vi "Get Local Chassis Modules References.vi"(8 "error in":errorcluster, 11 "Local Chassis Reference In":T1 format="%.0x") -> (0 "error out":errorcluster, 1 "Modules Found":bool, 2 "Modules References":T1[](array[typedef]) format="%.0x", 3 "Local Chassis Reference Out":T1 format="%.0x")   [LabVIEW 2017, in "Scan Engine Custom Device.lvlib"]
uses:
  Scan Engine Custom Device.lvlib
  <vilib>/NI Veristand/Custom Device API/Custom Device Item Ref.ctl
  Globals/Scan Engine GUIDs.vi
  <vilib>/NI Veristand/Custom Device Tools/Custom Device Utility Library/NI VeriStand - Search for All Items by GUID.vi
  <vilib>/NI Veristand/Custom Device Tools/Custom Device Utility Library/Custom Device Utility Library.lvlib
  <vilib>/NI Veristand/Custom Device API/Custom Device API.lvlib
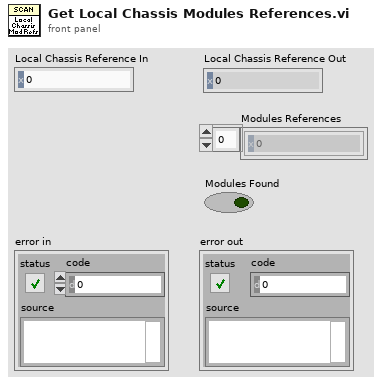
[diagram p1: front panel]
types:
  T1 = typedef "Custom Device API.lvlib/Custom Device Item Ref.ctl" = u64
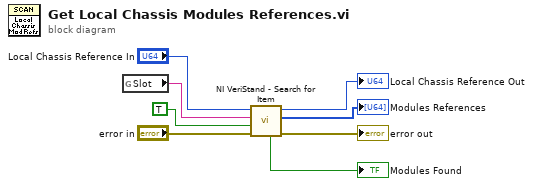
[diagram p0: block diagram]
diagram:
  n1 = global read "Scan Engine GUIDs.vi" "Slot"() -> (w8:string)
  n2 = call-poly <vilib>:"NI VeriStand - Search for Item.vi"("error in"="error in", "Find All? (T)"=TRUE, "Item GUID"=w8, "Section Ref in"="Local Chassis Reference In") -> ("error out"=→"error out":errorcluster, "Item Refs"=→"Modules References":T1[], "Section Ref out"=→"Local Chassis Reference Out":T1, "Found"=→"Modules Found":bool)  [unwired: 4 in]
